vi "Get Library Path.vi"() -> (3 "global library path":path)   [LabVIEW 2020, in "AIM ARINC 429 Hardware API.lvlib"]
uses:
  AIM ARINC 429 Hardware API.lvlib
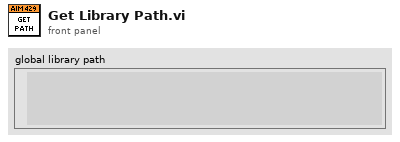
[diagram p1: front panel]
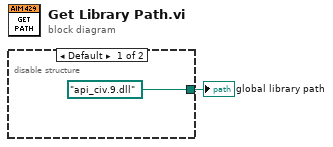
[diagram p0: block diagram]
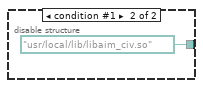
[diagram p2: hidden frame]
diagram:
  n1 = disable-structure shown="Default" {
    disable-tunnel: [path "api_civ.9.dll" ("GlobalDLLPath") path "/usr/local/lib/libaim_civ.so" ("DLL Path (if required)")] -> w1
    frame condition #0 (active) {
    }
    frame condition #1 {
    }
  }
  "global library path" <- w1
